vi "Set Pixels.vi"(8 "error in (no error)":errorcluster, 10 "Pixels":refnum<class "Pixel.lvclass">[][](array[class]), 11 "Image in":refnum<class "Image.lvclass">) -> (0 "error out":errorcluster, 3 "Image out":refnum<class "Image.lvclass">)   [LabVIEW 2020, in "RPI.SenseHat.Display.lvlib" / "Image.lvclass"]
doc: "Copies the Pixels array to image Pixels property. \n\nNote: Pixels is reshaped to the image length."
uses:
  Image.lvclass
  Pixel/Pixel.lvclass
  Image.lvclass/Image.ctl
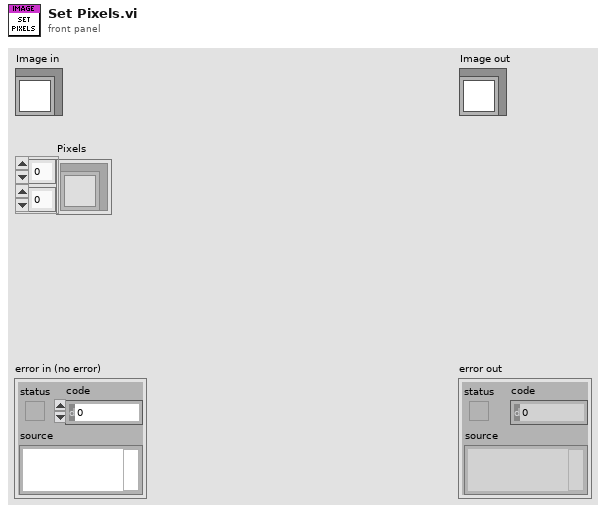
[diagram p1: front panel]
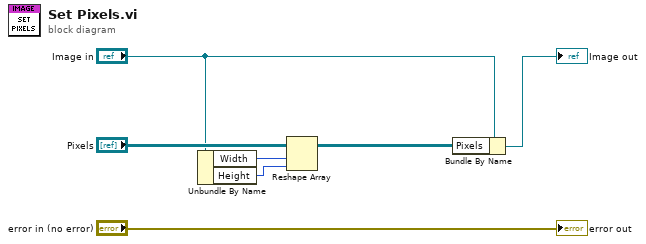
[diagram p0: block diagram]
diagram:
  n1 = Unbundle By Name("Image in") -> ("Width"=w2:i32, "Height"=w1:i32)
  n2 = Reshape Array("Pixels", w2, w1) -> (w3:refnum<class "Pixel.lvclass">[][])
  n3 = Bundle By Name(cluster="Image in", "Pixels"=w3) -> (→"Image out":refnum<class "Image.lvclass">)
  "error out" <- "error in (no error)"
